vi "AI engedélyezés.vi"(8 "error in (no error)":errorcluster, 11 "Message Queues":T1) -> (0 "error out":errorcluster, 3 "timeout in ms (-1)":i32)   [LabVIEW 2014]
uses:
  support/Message Queue/All Message Queues.ctl
  support/Message Queue/Message Cluster.ctl
  UI/UI data.ctl
  support/Message Queue/Message Queue.lvlib
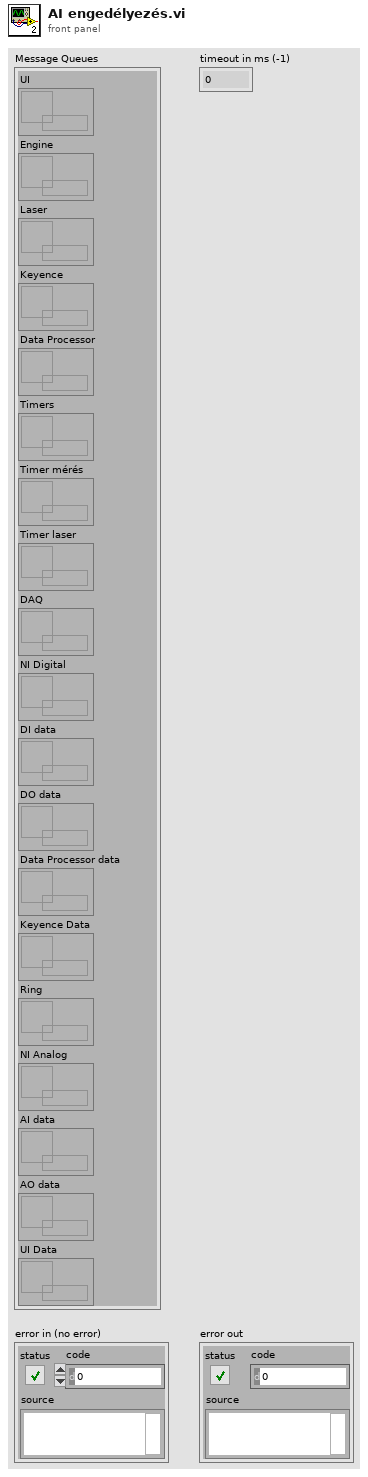
[diagram p1: front panel]
types:
  T1 = typedef "Message Queue.lvlib/All Message Queues.ctl" = cluster{"UI":refnum<queue>, "Engine":refnum<queue>, "Laser":refnum<queue>, "Keyence":refnum<queue>, "Data Processor":refnum<queue>, "Timers":refnum<queue>, "Timer mérés":refnum<queue>, "Timer laser":refnum<queue>, "DAQ":refnum<queue>, "NI Digital":refnum<queue>, "DI data":refnum<queue>, "DO data":refnum<queue>, "Data Processor data":refnum<queue>, "Keyence Data":refnum<queue>, "Ring":refnum<queue>, "NI Analog":refnum<queue>, "AI data":refnum<queue>, "AO data":refnum<queue>, "UI Data":refnum<queue>}
  T2 = typedef "UI data.ctl" = cluster{"AI engedélyezés":bool}
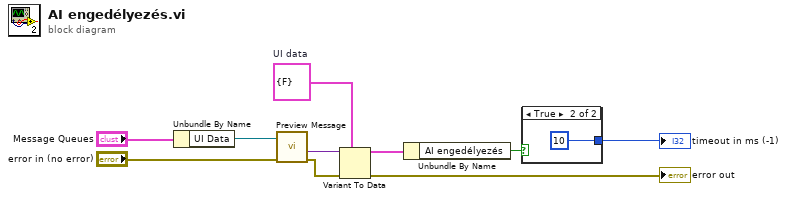
[diagram p0: block diagram]
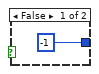
[diagram p2: hidden frame]
diagram:
  w7 = T2 {"AI engedélyezés"=FALSE}  # UI data
  n1 = Unbundle By Name("Message Queues") -> ("UI Data"=w2:refnum<queue>)
  n2 = call "Preview Message.vi"("error in (no error)"="error in (no error)", "Message Queue"=w2) -> ("error out"=w5:errorcluster, "Message Data"=w4:variant)  [unwired: 5 in, 3 out]
  n3 = Variant To Data(error in=w5, type=w7, Variant=w4) -> (data=w8:T2, error out=→"error out":errorcluster)
  n4 = Unbundle By Name(w8) -> ("AI engedélyezés"=w9:bool)
  n5 = case shown="True" w9 {
    tunnel: [-1 ("timeout in ms (-1)") 10 ("timeout in ms (-1)")] -> w10
    frame False {
    }
    frame True {
    }
  }
  "timeout in ms (-1)" <- w10
